vi "ThermoCouple_Packer.vi"(0 "dt":dbl, 5 "Temps in":dbl[](array[numeric]), 7 "Gradients in":dbl[](array[numeric]), 11 "Data in":cluster{"Temps":dbl[][], "Gradients":dbl[][]}) -> (4 "Temps":waveform(dbl)[](array[waveform]), 6 "Gradients":waveform(dbl)[](array[waveform]), 15 "Data out":cluster{"Temps":dbl[][], "Gradients":dbl[][]})   [LabVIEW 2020]
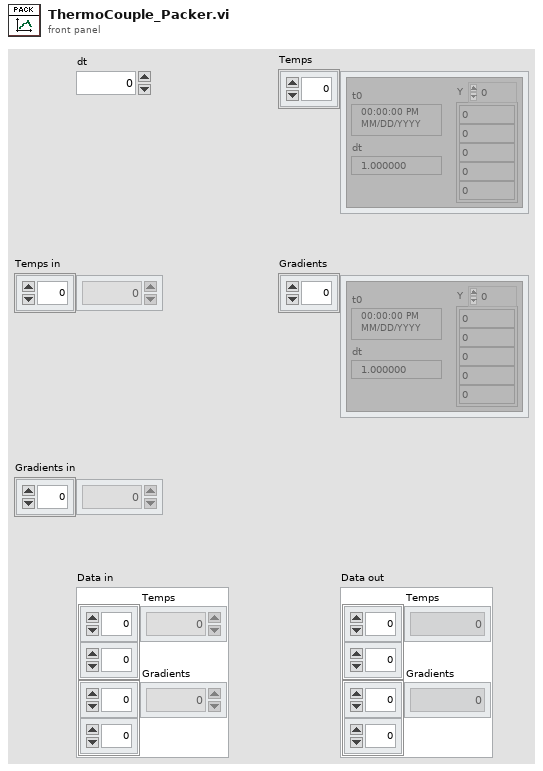
[diagram p1: front panel]
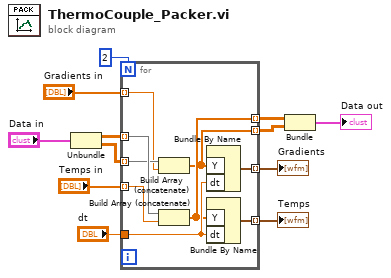
[diagram p0: block diagram]
diagram:
  n1 = Unbundle("Data in") -> ("Temps"=w4:dbl[][], "Gradients"=w3:dbl[][])
  n2 = for {
    N: 2 -> [_]
    tunnel: "Temps in" -> [w21] mode=indexing
    tunnel: w4 -> [w20] mode=indexing
    tunnel: "dt" -> [w17]
    tunnel: w3 -> [w19] mode=indexing
    tunnel: "Gradients in" -> [w18] mode=indexing
    tunnel: [w16] -> w12 mode=indexing
    tunnel: [w15] -> w11 mode=indexing
    tunnel: [w14] -> w6 mode=indexing
    tunnel: [w13] -> w7 mode=indexing
    n3 = Build Array (concatenate)(w19, w18) -> (w13:dbl[])
    n4 = Build Array (concatenate)(w20, w21) -> (w14:dbl[])
    n5 = Bundle By Name("Y"=w13, "dt"=w17) -> (w15:waveform(dbl))  [unwired: 1 in]
    n6 = Bundle By Name("Y"=w14, "dt"=w17) -> (w16:waveform(dbl))  [unwired: 1 in]
  }
  "Temps" <- w12
  "Gradients" <- w11
  n7 = Bundle(w6, w7) -> (→"Data out":cluster{dbl[][], dbl[][]})  [unwired: 1 in]
